vi "Drive Controller.vi"(8 "error in":errorcluster) -> ()   [LabVIEW 2017]
doc: "This VI executes continuously carrying out the current operation and responding to updates or new operation requests. It will often contain the timing or control code that is difficult to place directly in TeleOp. This VI generally opens all sensors and motors and isolates the rest of the robot code from knowing implementation details of how the operations are carried out."
uses:
  <vilib>/Rock Robotics/WPI/SafetyOutput/WPI_SafetyOutputConfigMenu.ctl
  <vilib>/Rock Robotics/WPI/ThirdParty/Sensors/navX/_TypeDefs/FRIC_navX_DeviceNumbersTypeDef.ctl
  <vilib>/addons/control/pid/NI_PID_pid.lvlib
  <vilib>/addons/control/pid/pid.llb/PID (DBL).vi
  <vilib>/Rock Robotics/SystemInterfaces/DIO/FPGA_DIOPWMChannel.ctl
  <vilib>/Rock Robotics/WPI/Counter/WPI_CounterDigitalInputToDigitalSource.vi
  <vilib>/Rock Robotics/SystemInterfaces/DIO/FPGA_DIOChannel.ctl
  Dawgma Programming Library/Controls/PurePursuit/RobotNeededPathData.ctl
  Drive Operations.ctl
  Drive Setpoints.ctl
  Configuration/Constants.vi
  Drive Published Globals.vi
  Framework/Robot Global Data.vi
  <vilib>/Rock Robotics/WPI/DriverStation/WPI_DriverStationRobotMode2.ctl
  <extravilib>/ChannelInstances/Lossy Stream-c(dbl,dbl,dbl,c(dbl,dbl)).lvlib
  <vilib>/Rock Robotics/Network Tables/NT Write Number.vi
  <vilib>/Rock Robotics/SystemInterfaces/i2clib/i2c_bus.ctl
  <vilib>/Rock Robotics/Network Tables/NT Read Number.vi
  <vilib>/Rock Robotics/WPI/RobotDrive/WPI_RobotDriveOpen2MotorWithSPARK.vi
  <vilib>/Rock Robotics/WPI/RobotDrive/WPI_RobotDriveOpen4MotorWithSPARK.vi
  <vilib>/Rock Robotics/WPI/Framework/Completion Status.ctl
panel:
  in  "MaxAccelDistance":dbl=170.0
  in  "MaxVelDistance":dbl=140.0
  in  "MaxAccelAngle":dbl
  in  "MaxVelAngle":dbl
  in  "TurnToAngleGains":T1={"FFV"=0.0032, "FFA"=0.0, "Vel PID"={"P"=0.0, "I"=0.0, "D"=0.0}} {"Vel PID"."D" format="%.3f"; "Vel PID"."I" format="%.3f"; "Vel PID"."P" format="%.3f"}
  in  "PixyCenteringValues":cluster{"X":dbl, "Y":dbl}[](array[cluster])=[{"X"=0.0, "Y"=70.0}, {"X"=70.0, "Y"=100.0}]
  in  "EndCondArea":i32=11000
  in  "MaxY":i32=130
  in  "KpY":dbl=0.0001
  in  "KpX":dbl=0.1
  in  "MaxSpeed":dbl=0.3
  in  "KdX":dbl=0.07
  in  "AreaSetpoint":i32
  in  "CenterSetpoint":i32=80
  out "Numeric":dbl=4.0
  out "Yaw 2":dbl=-45.089999999999996
  in  "Gains":T1={"FFV"=0.0059, "FFA"=0.0019, "Vel PID"={"P"=0.01, "I"=0.0, "D"=0.0}}
  in  "Interactive Values":T2={"Operation"=enum."Turn to Angle", "Left Speed"=-0.27, "Right Speed"=0.27, "Duration"=2.0, "Speed"=0.0, "Start Angle"=0.0, "Target Angle"=180.0, "Distance (inch)"=0.0, "Start Point (inch)"=0.0, "RobotNeededPathData"={"Path"=[], "MaxVel"=0.0, "MaxAccel"=-1.0, "Backwards?"=FALSE, "PointSpacing"=0.0, "LookaheadDist"=0.0, "Speed/Curve"=1.8, "SlowDistanceAtEnd"=12.0, "SlowSpeed"=15.0, "MaxDeAccel"=0.0}, "Start Point 2"=0.0} {"RobotNeededPathData"."SlowSpeed" format="%#_13g"; "RobotNeededPathData"."SlowDistanceAtEnd" format="%#_13g"; "RobotNeededPathData"."Speed/Curve" format="%#_13g"}
  in  "Buttons":cluster{"Execute Cmd":bool, "Abort Cmd":bool}
  out "Command Timing":cluster{"Start Time (ms)":u32, "Iterations":i32}={"Start Time (ms)"=372507, "Iterations"=0}
  out "Status":T5
  out "Setpoints":T6(graph)
  out "Current\nCmd":string="Started at  14:51:47.884\nDefault: Reserve,  L 0.0, R 0.0, D 0.000000"
  # "Tip: The graph shows the motor setpoints. It may also be helpful to observe inputs and sensor values.\nYou may also want to display tuning or debugging controls."
  # ".0088"
  # ".0017"
  # ".02"
  # "Interactive Command: You may fill in the settings for a command\nand schedule it with the Execute button. You can observe and abort\nany command while fine tuning the code for the controller."
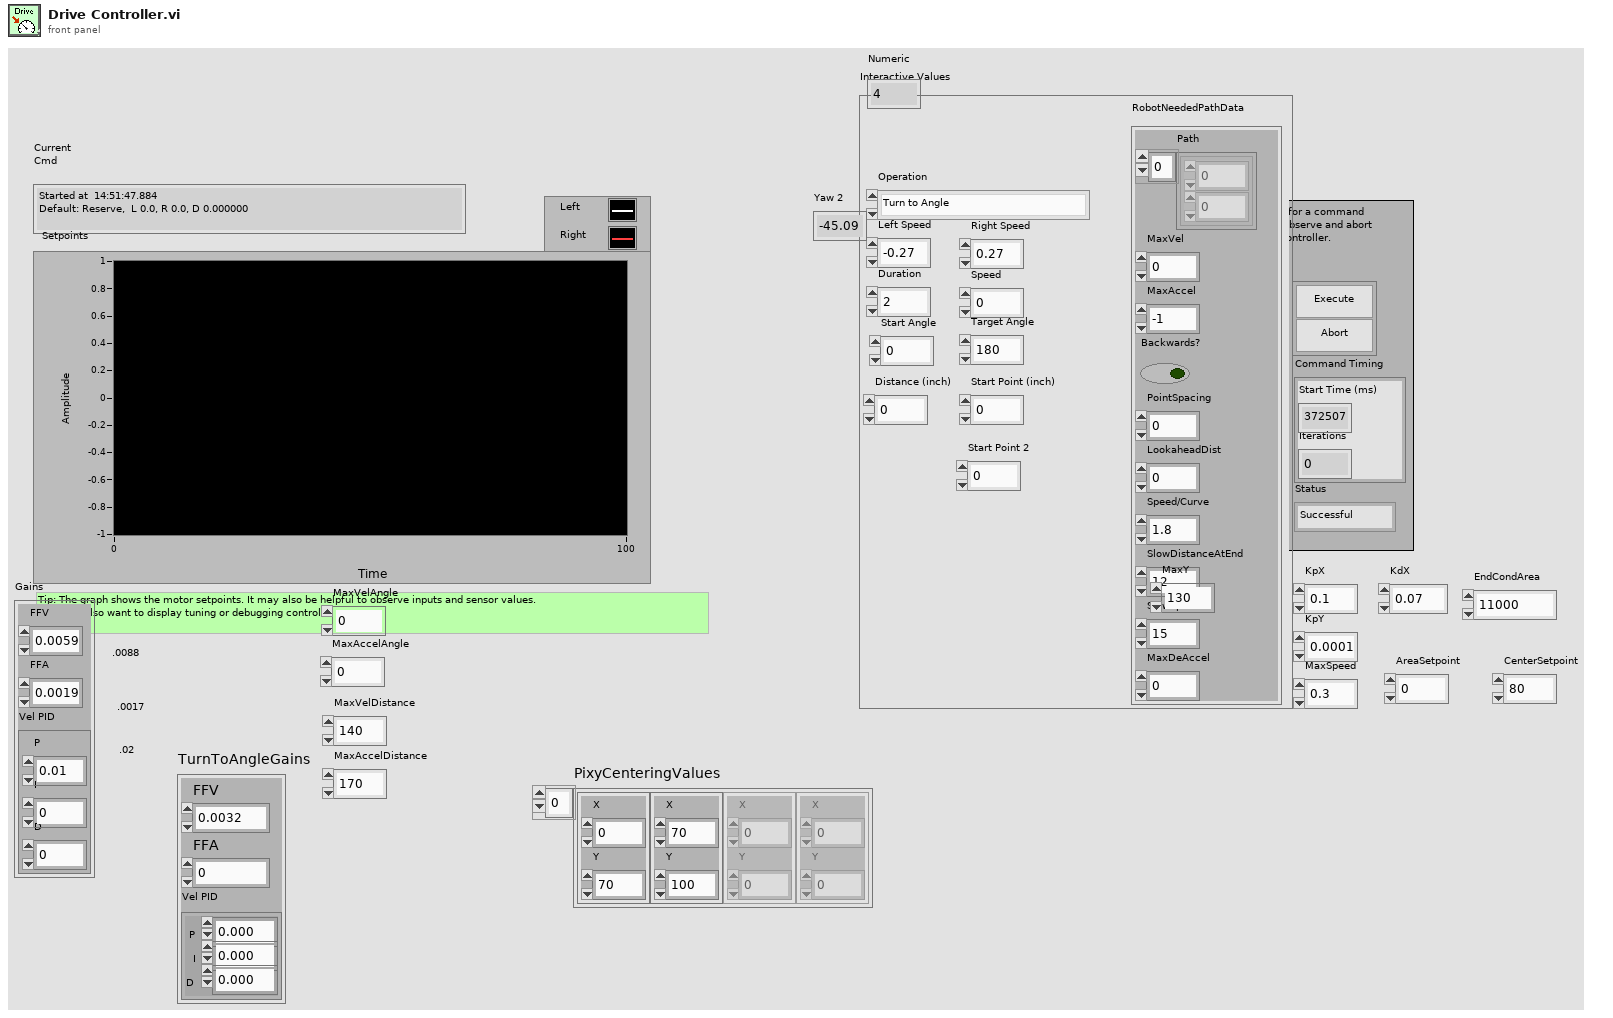
[diagram p1: front panel]
types:
  T1 = cluster{"FFV":dbl, "FFA":dbl, "Vel PID":cluster{"P":dbl, "I":dbl, "D":dbl}}
  T2 = typedef "Drive Setpoints.ctl" = cluster{"Operation":T3, "Left Speed":dbl, "Right Speed":dbl, "Duration":dbl, "Speed":dbl, "Start Angle":dbl, "Target Angle":dbl, "Distance (inch)":dbl, "Start Point (inch)":dbl, "RobotNeededPathData":T4, "Start Point 2":dbl}
  T3 = typedef "Drive Operations.ctl" = enum16{"Reserve", "Read Current", "Immediate", "Drive for Time", "Drive for Distance", "Turn to Angle", "Arc Turn", "Drive Path", "Drive To Cube"}
  T4 = typedef "RobotNeededPathData.ctl" = cluster{"Path":cluster{dbl, dbl}[], "MaxVel":dbl, "MaxAccel":dbl, "Backwards?":bool, "PointSpacing":dbl, "LookaheadDist":dbl, "Speed/Curve":dbl, "SlowDistanceAtEnd":dbl, "SlowSpeed":dbl, "MaxDeAccel":dbl}
  T5 = typedef "Completion Status.ctl" = enum16{"Successful", "Aborted", "Incomplete"}
  T6 = cluster{"Left Setpoint":dbl, "Right Setpoint":dbl}
  T7 = typedef "i2c_bus.ctl" = enum16{"I2C On-Board", "I2C MXP", "Invalid"}
  T8 = typedef "FPGA_DIOChannel.ctl" = enum8{"DIO 0", "DIO 1", "DIO 2", "DIO 3", "DIO 4", "DIO 5", "DIO 6", "DIO 7", "DIO 8", "DIO 9", "DIO MXP 0", "DIO MXP 1", "DIO MXP 2", "DIO MXP 3", "DIO MXP 4", "DIO MXP 5", "DIO MXP 6", "DIO MXP 7", "DIO MXP 8", "DIO MXP 9", "DIO MXP 10", "DIO MXP 11", "DIO MXP 12", "DIO MXP 13", "DIO MXP 14", "DIO MXP 15", "SPI Port CS1", "SPI Port CS2", "SPI Port CS3", "SPI Port MISO", "SPI Port MOSI", "Invalid"}
  T9 = typedef "FPGA_DIOPWMChannel.ctl" = enum8{"PWM 0", "PWM 1", "PWM 2", "PWM 3", "PWM 4", "PWM 5", "PWM 6", "PWM 7", "PWM 8", "PWM 9", "PWM MXP 0", "PWM MXP 1", "PWM MXP 2", "PWM MXP 3", "PWM MXP 4", "PWM MXP 5", "PWM MXP 6", "PWM MXP 7", "PWM MXP 8", "PWM MXP 9", "Invalid"}
  T10 = typedef "WPI_SafetyOutputConfigMenu.ctl" = enum16{"Enable", "Disable"}
  T11 = typedef "WPI_DigitalInputDevRef.ctl" = cluster{"DevStatus":errorcluster, "DIO Channel":T8}
  T12 = typedef "FPGA_CounterEncoderSourceConvertionLVSourceType.ctl" = cluster{"DevStatus":errorcluster, "AnalogTriggerMode?":bool, "DigitalMode":cluster{"DIO Channel":T13}, "AnalogTriggerMode":cluster{"AnalogTriggerIndex":T14, "OutputType":T15}}
  T13 = typedef "FPGA_DIODigitalSourceChannel.ctl" = enum8{"DIO 0", "DIO 1", "DIO 2", "DIO 3", "DIO 4", "DIO 5", "DIO 6", "DIO 7", "DIO 8", "DIO 9", "DIO MXP 0", "DIO MXP 1", "DIO MXP 2", "DIO MXP 3", "DIO MXP 4", "DIO MXP 5", "DIO MXP 6", "DIO MXP 7", "DIO MXP 8", "DIO MXP 9", "DIO MXP 10", "DIO MXP 11", "DIO MXP 12", "DIO MXP 13", "DIO MXP 14", "DIO MXP 15", "Disabled"}
  T14 = typedef "FPGA_AnalogTriggerIndex.ctl" = enum8{"Trig 0", "Trig 1", "Trig 2", "Trig 3", "Trig 4", "Trig 5", "Trig 6", "Trig 7", "Invalid"}
  T15 = typedef "FPGA_AnalogTriggerOutType.ctl" = enum16{"InWindow", "TriggerState", "Rising", "Falling"}
  T16 = typedef "WPI_EncoderDevRef.ctl" = cluster{"DevStatus":errorcluster, "EncoderIndex":T17, "CounterIndex":T18, "DistancePerCount":dbl, "Decoding Type":T19}
  T17 = typedef "FPGA_EncoderIdx.ctl" = enum8{"Enc 0", "Enc 1", "Enc 2", "Enc 3", "Enc 4", "Enc 5", "Enc 6", "Enc 7", "Invalid"}
  T18 = typedef "FPGA_CounterCtrSystemIndex.ctl" = enum8{"Ctr 0", "Ctr 1", "Ctr 2", "Ctr 3", "Ctr 4", "Ctr 5", "Ctr 6", "Ctr 7", "Invalid"}
  T19 = typedef "WPI_EncoderType.ctl" = enum16{"1x", "2x", "4x"}
  T20 = typedef "WPI_RobotDriveDevRef.ctl" = cluster{"DevStatus":errorcluster, "Motors[]":T21[], "Square Inputs":bool, "Max Output":dbl}
  T21 = typedef "WPI_MotorControlDeviceRef.ctl" = cluster{"DeviceStatus":errorcluster, "Type":T22, "PWM":cluster{"PWM Channel":T9, "DeadBand":T23}, "CAN":cluster{"Device Number":u8, "SetOutput VI Ref":variant, "GetOutput VI Ref":variant, "Enable VI Ref":variant, "Disable VI Ref":variant, "Data":variant}, "Invert":bool, "DIO PWM":cluster{"PWM \"Enable\" Channel":T9, "DIOChannel":T8, "PWM Rate":dbl}}
  T22 = typedef "WPI_MotorControlType.ctl" = enum16{"PWM", "CAN", "DIO PWM"}
  T23 = typedef "WPI_PWMDeadband.ctl" = cluster{"Name":string, "maxPositivePwm":i32, "minPositivePwm":i32, "centerPwm":i32, "maxNegativePwm":i32, "minNegativePwm":i32, "angularRange":u16}
  T24 = typedef "WPI_I2CDevRef.ctl" = cluster{"DevStatus":errorcluster, "Device Address":u8, "Handle":i32, "I2C Bus":T7}
  T25 = typedef "Command Status Info.ctl" = cluster{"Name":string, "Status":T5, "notifier out":T26}
  T26 = typedef "Completion Notifier.ctl" = refnum<notifier>
  T27 = cluster{"SubSystem Data":T2, cluster{"Start Time (ms)":u32, "Iterations":i32}, cluster{"Command Info":T25, "Description":string, "Default Command":T2, "queue out":refnum<queue>, "Subsystem Name":string}}
  T28 = cluster{"X":i32, "Y":i32, "Width":i32, "Height":i32, "ValidData":bool, "Timestamp":u32}
  T29 = typedef "WPI_DriverStationRobotMode2.ctl" = enum16{"Autonomous Disabled", "Autonomous Enabled", "Teleop Disabled", "Teleop Enabled", "Disconnected", "Finish", "Test Disabled", "Test Enabled", "Emergency Stopped"}
  T30 = cluster{"Yaw":dbl, "Roll":dbl, "Pitch":dbl, "Heading":dbl, "Fused Heading":dbl}
  T31 = cluster{"dx/dt":dbl, "dx/dt":dbl, dbl, cluster{dbl, dbl}}
  T32 = typedef "Lossy Stream-c(dbl,dbl,dbl,c(dbl,dbl)).lvlib/)Channel.ctl" = refnum<queue>
  T33 = cluster{"LeftDistance":dbl, "RightDistance":dbl, "LeftVelocity":dbl, "RightVelocity":dbl, "Angle":dbl, "Location":cluster{dbl, dbl}}
  T34 = typedef "FRIC_navX_DeviceNumbersTypeDef.ctl" = enum16{"Dev0", "Dev1", "Dev2", "Dev3"}
  T35 = cluster{"proportional gain (Kc)":dbl, "integral time (Ti, min)":dbl, "derivative time (Td, min)":dbl}
  T36 = cluster{"dx/dt":dbl, "dx/dt":dbl, "Yaw":dbl, cluster{dbl, dbl}}
  T37 = cluster{"SubSystem Data":T2, cluster{"Start Time (ms)":u32, "Iterations":i32}, "Default Command Arguments":cluster{"Command Info":T25, "Description":string, "Default Command":T2, "queue out":refnum<queue>, "Subsystem Name":string}}
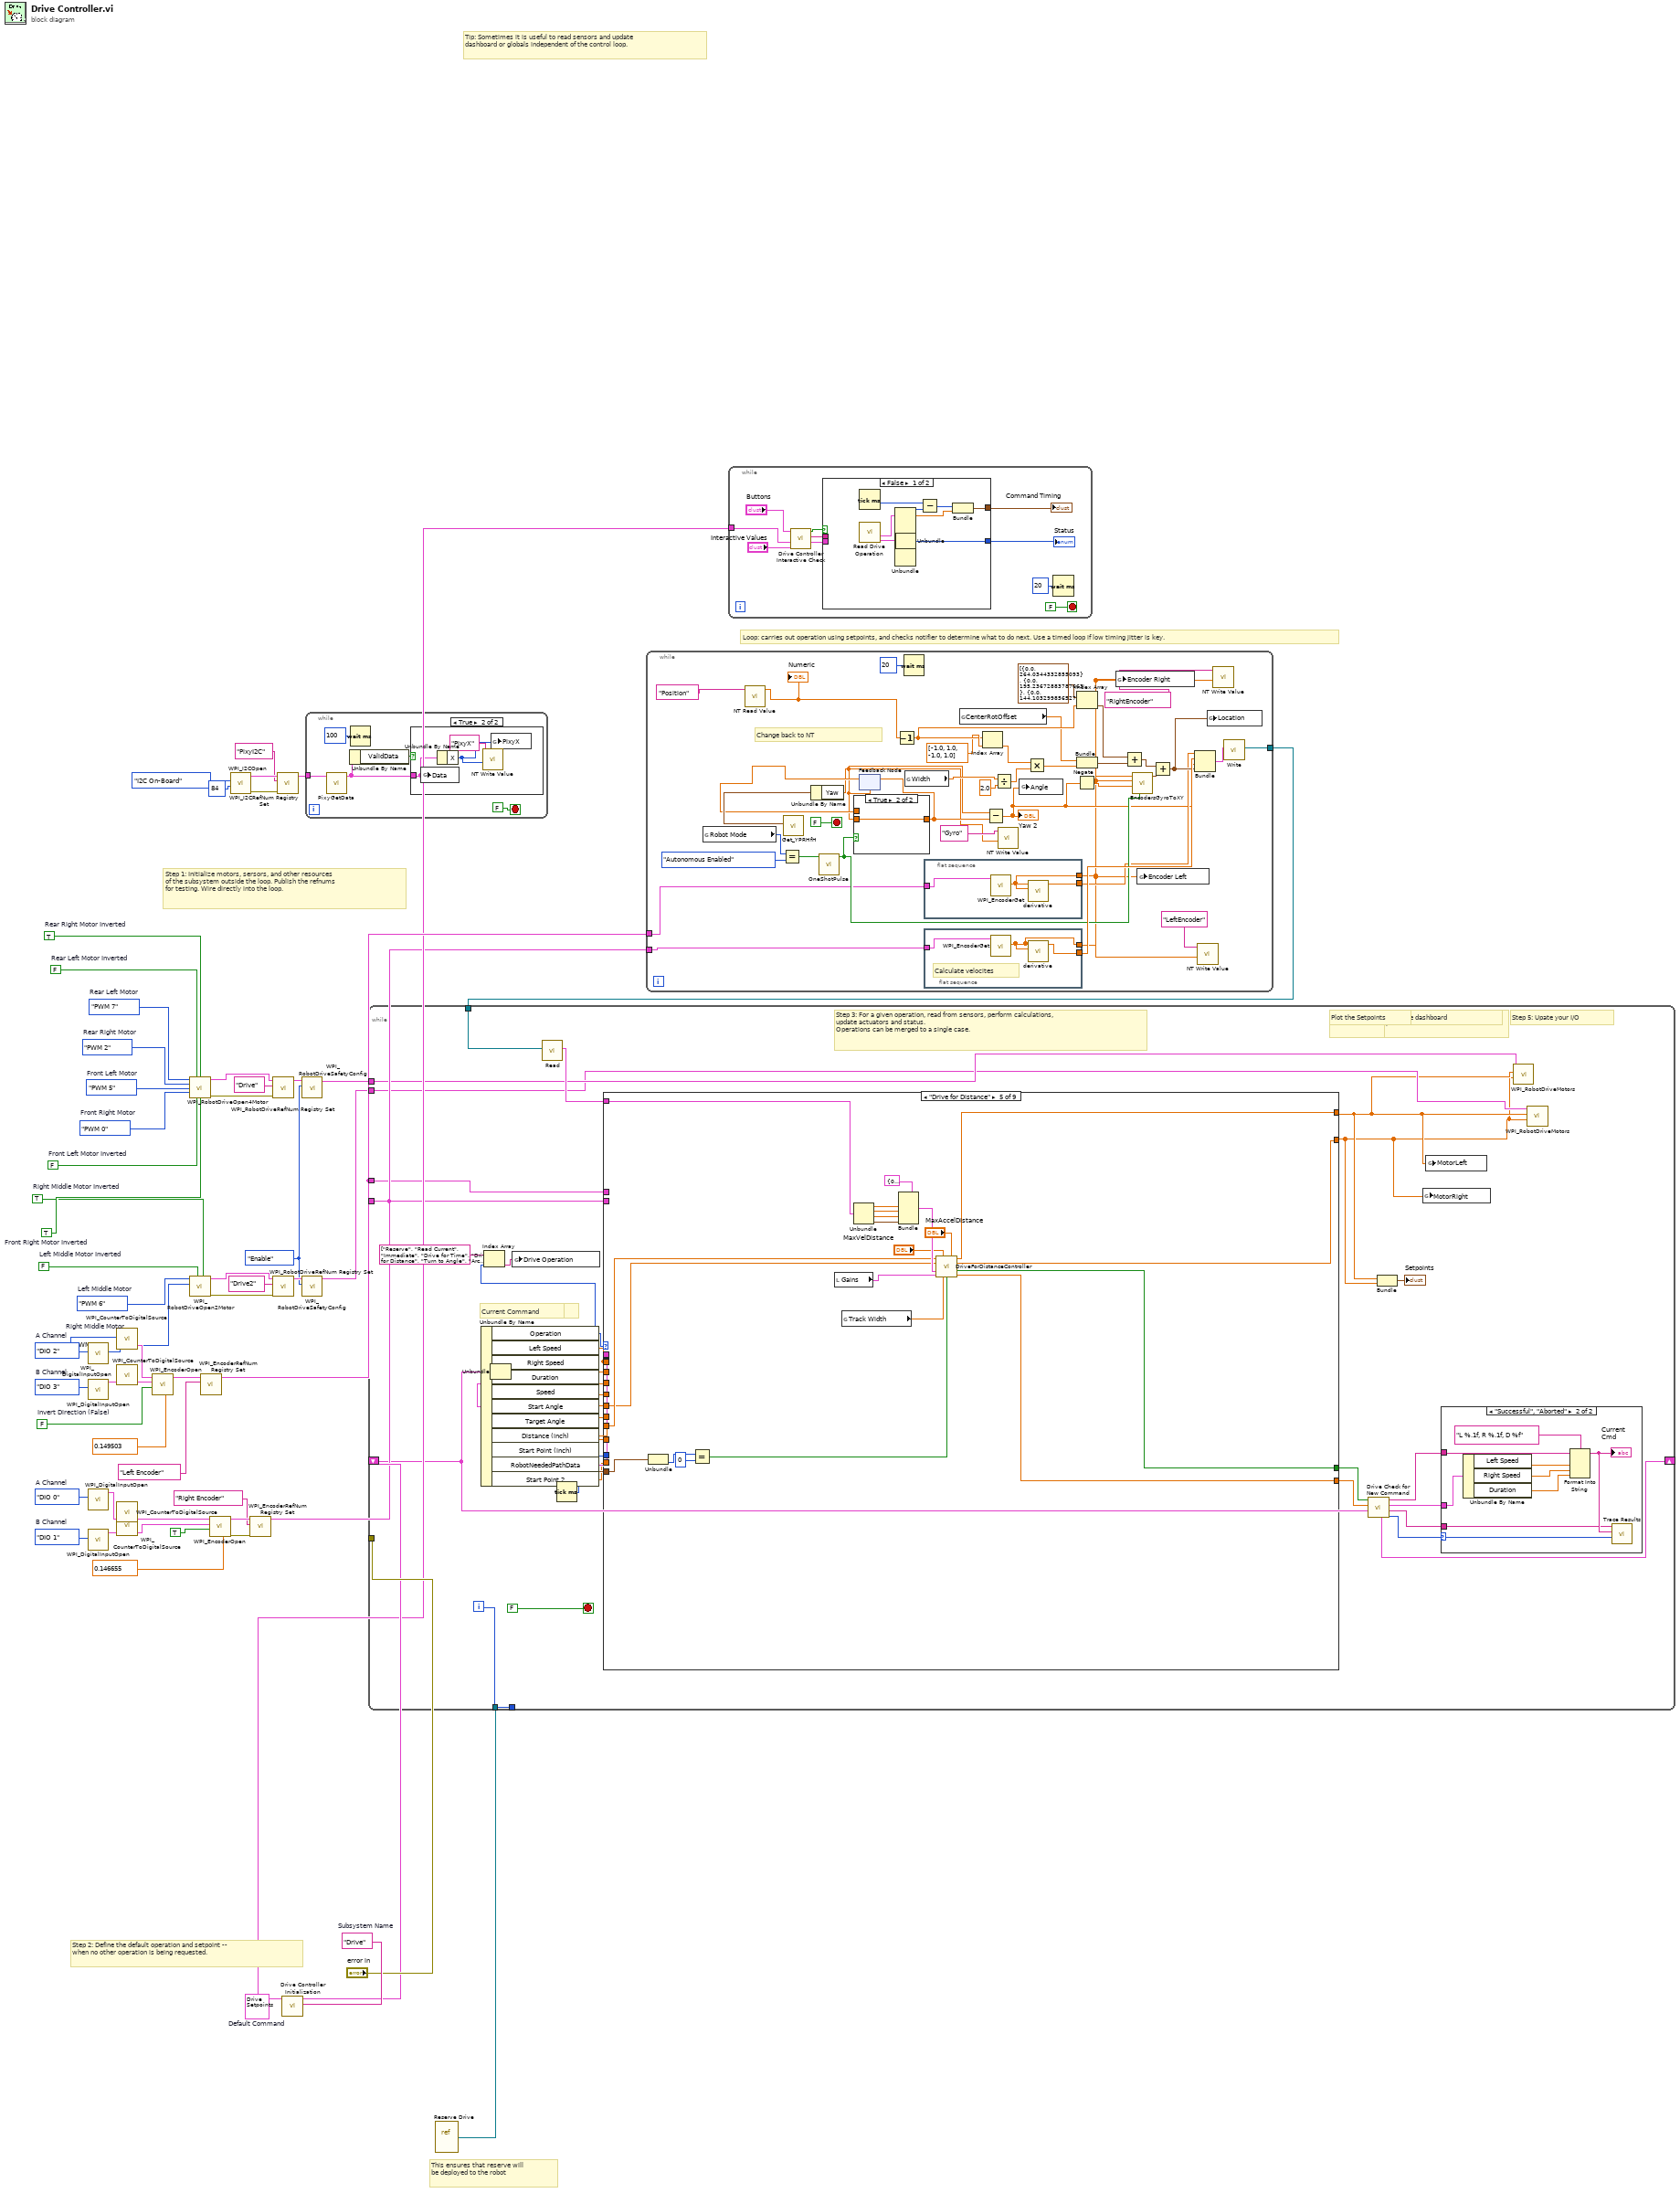
[diagram p0: block diagram]
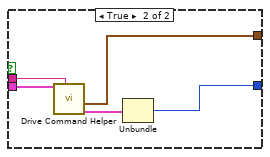
[diagram p4: hidden frame]
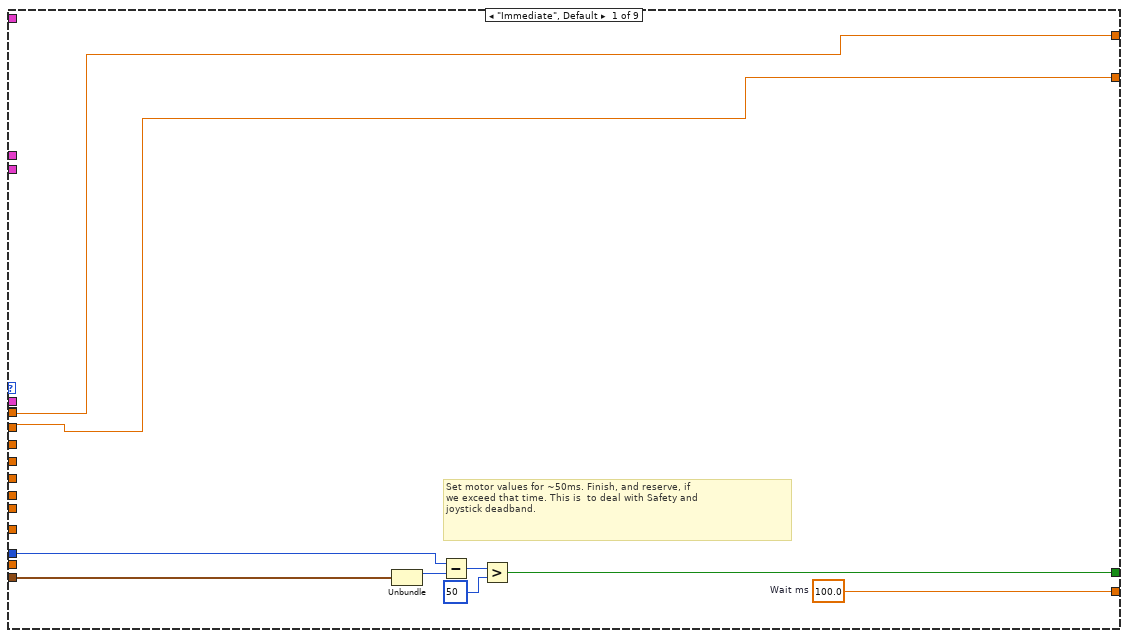
[diagram p5: hidden frame]
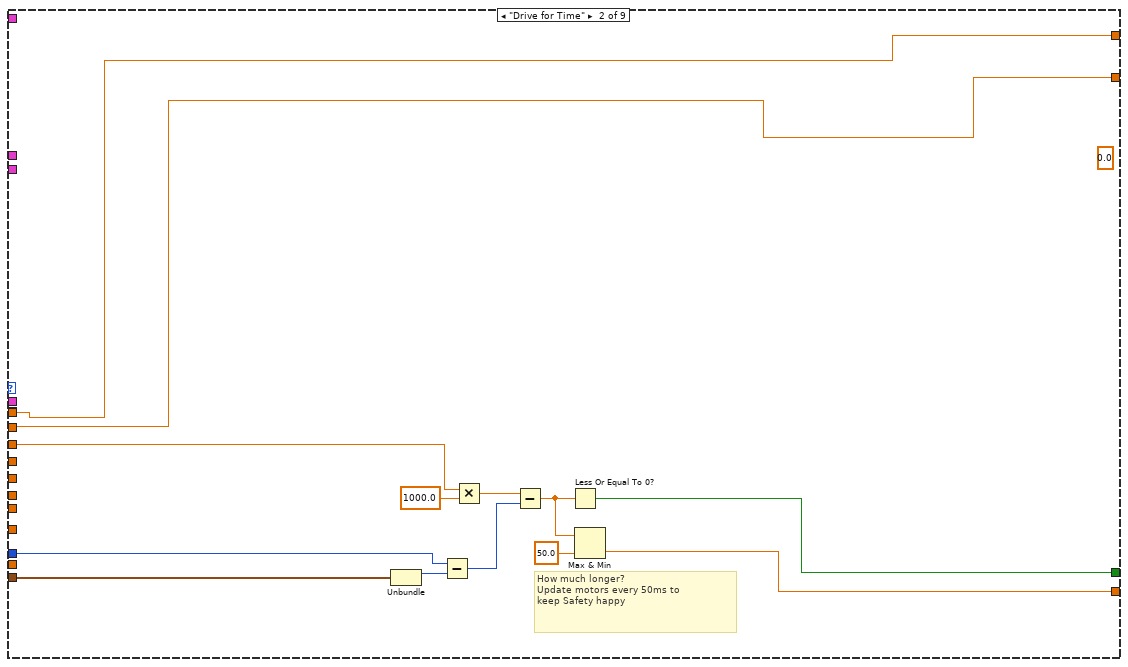
[diagram p6: hidden frame]
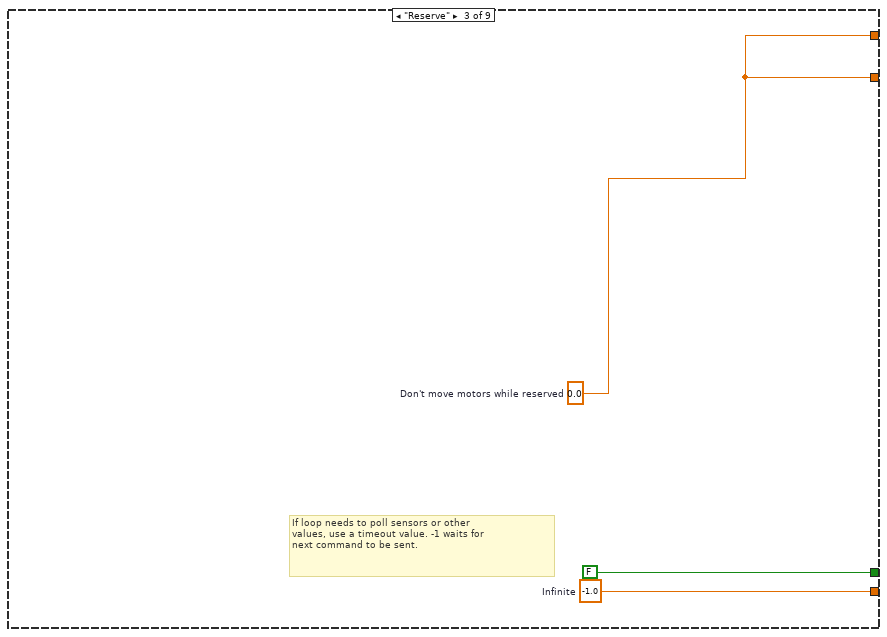
[diagram p7: hidden frame]
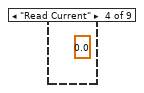
[diagram p8: hidden frame]
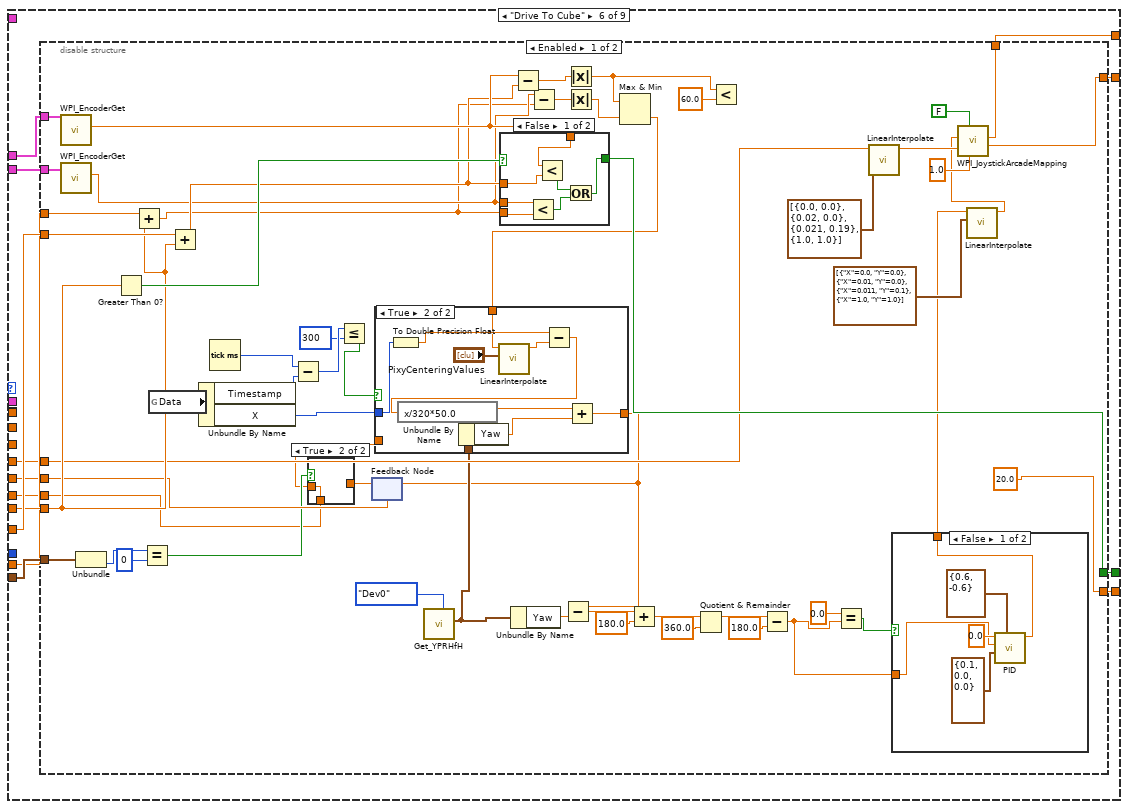
[diagram p9: hidden frame]
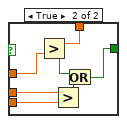
[diagram p12: hidden frame]
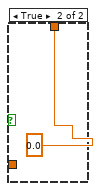
[diagram p13: hidden frame]
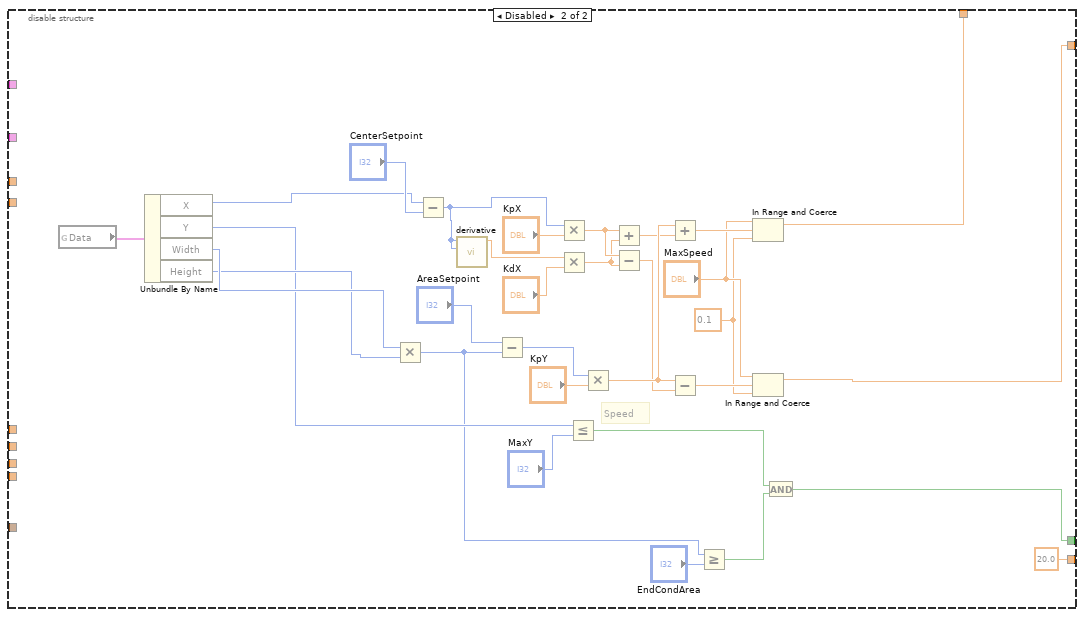
[diagram p14: hidden frame]
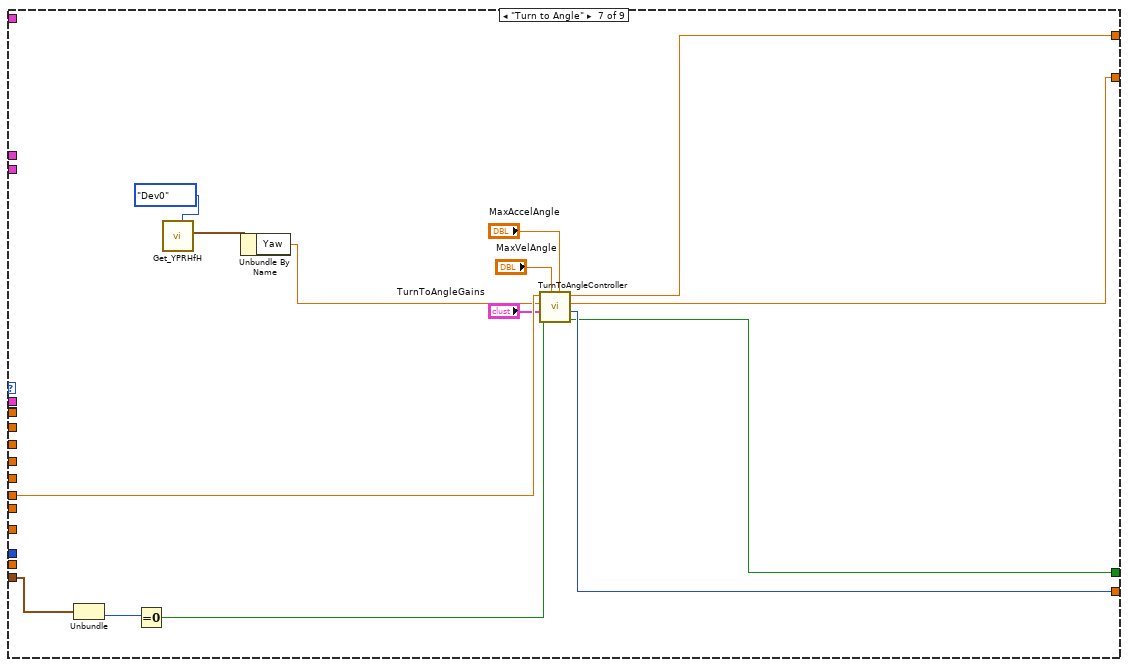
[diagram p15: hidden frame]
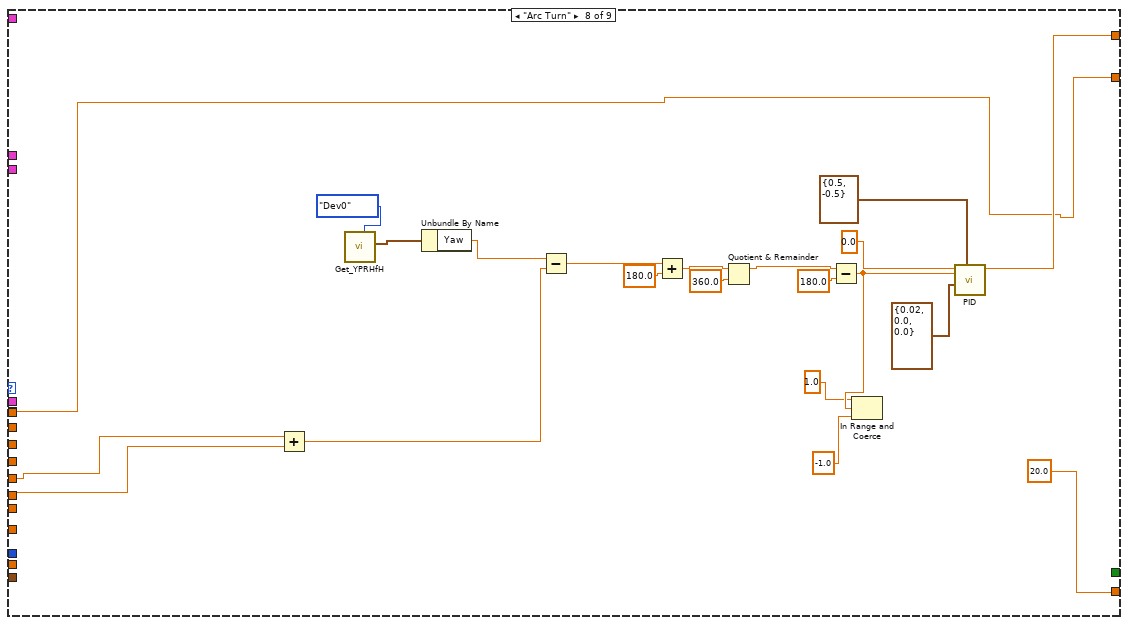
[diagram p16: hidden frame]
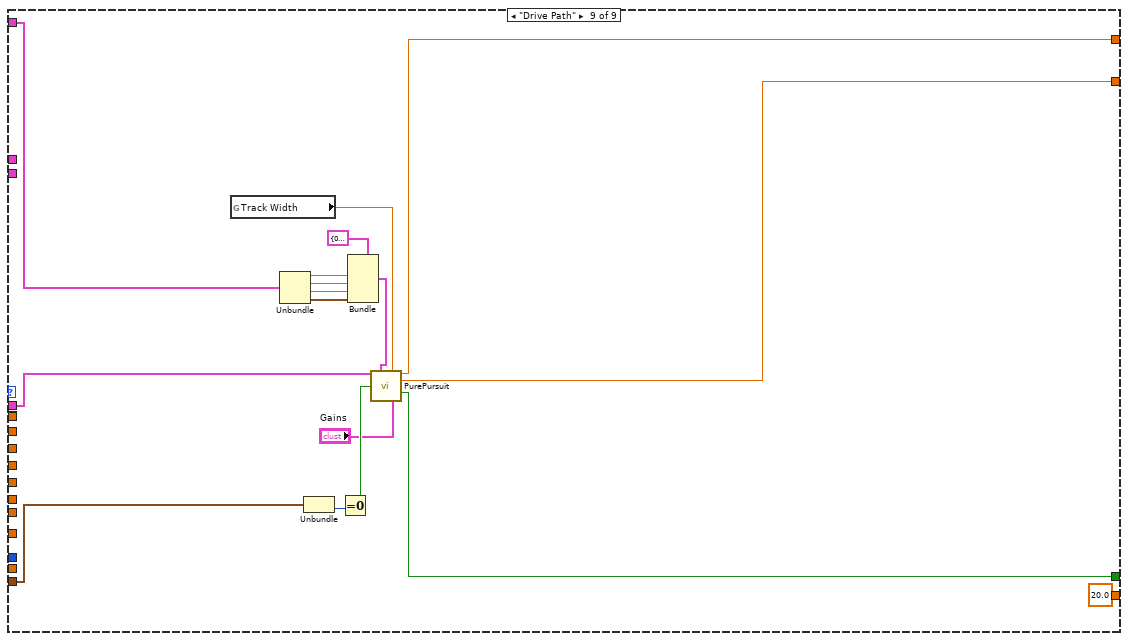
[diagram p17: hidden frame]
diagram:
  w10 = FPGA_DIOChannel."DIO 1"  # B Channel
  w13 = FPGA_DIOChannel."DIO 0"  # A Channel
  w20 = T2 {"Operation"=enum."Reserve", "Left Speed"=0.0, "Right Speed"=0.0, "Duration"=0.0, "Speed"=0.0, "Start Angle"=0.0, "Target Angle"=0.0, "Distance (inch)"=0.0, "Start Point (inch)"=0.0, "RobotNeededPathData"={"Path"=[], "MaxVel"=0.0, "MaxAccel"=0.0, "Backwards?"=FALSE, "PointSpacing"=0.0, "LookaheadDist"=0.0, "Speed/Curve"=1.8, "SlowDistanceAtEnd"=12.0, "SlowSpeed"=15.0, "MaxDeAccel"=0.0}, "Start Point 2"=0.0}  # Default Command
  w27 = TRUE  # Right Middle Motor Inverted
  w28 = FALSE  # Left Middle Motor Inverted
  w31 = FPGA_DIOPWMChannel."PWM 1"  # Right Middle Motor
  w32 = FPGA_DIOPWMChannel."PWM 6"  # Left Middle Motor
  w41 = FALSE  # Invert Direction (False)
  w34 = FPGA_DIOChannel."DIO 3"  # B Channel
  w35 = FPGA_DIOChannel."DIO 2"  # A Channel
  w43 = TRUE  # Front Right Motor Inverted
  w44 = FALSE  # Front Left Motor Inverted
  w45 = TRUE  # Rear Right Motor Inverted
  w46 = FALSE  # Rear Left Motor Inverted
  w47 = FPGA_DIOPWMChannel."PWM 0"  # Front Right Motor
  w48 = FPGA_DIOPWMChannel."PWM 5"  # Front Left Motor
  w49 = FPGA_DIOPWMChannel."PWM 2"  # Rear Right Motor
  w50 = FPGA_DIOPWMChannel."PWM 7"  # Rear Left Motor
  w22 = WPI_SafetyOutputConfigMenu."Enable" ("mode")
  w58 = "Drive"  # Subsystem Name
  # "Step 1: Initialize motors, sersors, and other resources\nof the subsystem outside the loop. Publish the refnums\nfor testing. Wire directly into the loop."
  # "Step 2: Define the default operation and setpoint --\nwhen no other operation is being requested."
  # "This ensures that reserve will\nbe deployed to the robot"
  # "Tip: Sometimes it is useful to read sensors and update\ndashboard or globals independent of the control loop."
  # "Loop: carries out operation using setpoints, and checks notifier to determine what to do next. Use a timed loop if low timing jitter is key."
  n1 = call <vilib>:"WPI_DigitalInputOpen.vi"("DIO Channel"=w35) -> ("DigitalInputDevRef"=w38:T11)  [unwired: 1 in, 9 out]
  n2 = call <vilib>:"WPI_DigitalInputOpen.vi"("DIO Channel"=w34) -> ("DigitalInputDevRef"=w37:T11)  [unwired: 1 in, 9 out]
  n3 = call <vilib>:"WPI_DigitalInputOpen.vi"("DIO Channel"=w13) -> ("DigitalInputDevRef"=w14:T11)  [unwired: 1 in, 9 out]
  n4 = call <vilib>:"WPI_DigitalInputOpen.vi"("DIO Channel"=w10) -> ("DigitalInputDevRef"=w11:T11)  [unwired: 1 in, 9 out]
  n5 = call-poly <vilib>:"WPI_CounterToDigitalSource.vi"("DigitalInputDevRef"=w38) -> ("Digital Source"=w39:T12)  [unwired: 6 out]
  n6 = call-poly <vilib>:"WPI_CounterToDigitalSource.vi"("DigitalInputDevRef"=w37) -> ("Digital Source"=w36:T12)  [unwired: 6 out]
  n7 = call-poly <vilib>:"WPI_CounterToDigitalSource.vi"("DigitalInputDevRef"=w14) -> ("Digital Source"=w15:T12)  [unwired: 6 out]
  n8 = call-poly <vilib>:"WPI_CounterToDigitalSource.vi"("DigitalInputDevRef"=w11) -> ("Digital Source"=w12:T12)  [unwired: 6 out]
  n9 = call <vilib>:"WPI_EncoderOpen.vi"("DistancePerCount"=0.149503, "Invert Direction (False)"=w41, "BSource"=w36, "ASource"=w39) -> ("EncoderDevRef"=w40:T16)  [unwired: 4 in, 3 out]
  n10 = call-poly <vilib>:"WPI_RobotDriveOpen4Motor.vi"("Rear Left Motor"=w50, "Rear Left Motor Inverted"=w46, "Rear Right Motor Inverted"=w45, "Rear Right Motor"=w49, "Front Left Motor"=w48, "Front Right Motor"=w47, "Front Left Motor Inverted"=w44, "Front Right Motor Inverted"=w43) -> ("RobotDriveDevRef"=w57:T20, "error out"=w55:errorcluster)  [unwired: 6 in]
  n11 = call-poly <vilib>:"WPI_RobotDriveOpen2Motor.vi"("Right Motor Inverted"=w27, "Left Motor Inverted"=w28, "Right Motor"=w31, "Left Motor"=w32) -> ("error out"=w26:errorcluster, "RobotDriveDevRef"=w30:T20)  [unwired: 6 in]
  n12 = call <vilib>:"WPI_EncoderRefNum Registry Set.vi"("refnum name"="Left Encoder", "EncoderDevRef"=w40) -> ("EncoderDevRef"=w33:T16)  [unwired: 8 in, 1 out]
  n13 = call <vilib>:"WPI_EncoderOpen.vi"("DistancePerCount"=0.146655, "Invert Direction (False)"=TRUE, "BSource"=w12, "ASource"=w15) -> ("error out"=w17:errorcluster, "EncoderDevRef"=w16:T16)  [unwired: 4 in, 2 out]
  n14 = call <vilib>:"WPI_I2COpen.vi"("Device Address"=u8 84, "I2C Bus"=i2c_bus."I2C On-Board") -> ("error out"=w3:errorcluster, "I2CDevRef"=w4:T24)  [unwired: 8 in]
  n15 = call <vilib>:"WPI_EncoderRefNum Registry Set.vi"("error in (no error)"=w17, "refnum name"="Right Encoder", "EncoderDevRef"=w16) -> ("EncoderDevRef"=w18:T16)  [unwired: 7 in, 1 out]
  n16 = call <vilib>:"WPI_RobotDriveRefNum Registry Set.vi"("error in (no error)"=w55, "refnum name"="Drive", "RobotDriveDevRef"=w57) -> ("RobotDriveDevRef"=w25:T20)  [unwired: 1 in, 7 out]
  n17 = call <vilib>:"WPI_RobotDriveRefNum Registry Set.vi"("error in (no error)"=w26, "refnum name"="Drive2", "RobotDriveDevRef"=w30) -> ("RobotDriveDevRef"=w24:T20)  [unwired: 7 in, 1 out]
  n18 = call <vilib>:"WPI_I2CRefNum Registry Set.vi"("error in (no error)"=w3, "refnum name"="PixyI2C", "I2CDevRef"=w4) -> ("I2CDevRef"=w1:T24)  [unwired: 7 in, 1 out]
  n19 = call "Drive Controller Initialization.vi"("Subsystem Name"=w58, "Default Command"=w20) -> ("Current Command"=w52:T27)  [unwired: 9 in]
  n20 = call <vilib>:"WPI_RobotDriveSafetyConfig.vi"("mode"=w22, "RobotDriveDevRef"=w25) -> ("RobotDriveDevRef"=w54:T20)  [unwired: 8 in, 1 out]
  n21 = call <vilib>:"WPI_RobotDriveSafetyConfig.vi"("mode"=w22, "RobotDriveDevRef"=w24) -> ("RobotDriveDevRef"=w23:T20)  [unwired: 8 in, 1 out]
  n22 = while {
    tunnel: w1 -> [w62]
    stop <- FALSE stop-if-true
    n23 = call "PixyGetData.vi"("I2CDevRef"=w62) -> ("Data"=w61:T28)  [unwired: 10 in]
    n24 = Unbundle By Name(w61) -> ("ValidData"=w60:bool)
    n25 = Wait (ms)(milliseconds to wait=u32 100) -> ()  [unwired: 1 out]
    n26 = case shown="True" w60 {
      tunnel: w61 -> [_ w66]
      frame False {
      }
      frame True {
        n27 = global write "Drive Published Globals.vi" "Data"(w66) -> ()
        n28 = Unbundle By Name(w66) -> ("X"=w64:i32)
        n29 = call-poly <vilib>:"NT Write Value.vi"("Numeric"=w64, "Name"="PixyX") -> ()  [unwired: 9 in, 1 out]
        n30 = global write "Drive Published Globals.vi" "PixyX"(w64) -> ()
      }
    }
  }
  n31 = vi-ref "Reserve Drive.vi"() -> (w51:refnum<vi>)
  n32 = while {
    tunnel: [w78] -> w19
    tunnel: w18 -> [w77]
    tunnel: w33 -> [w76]
    stop <- FALSE stop-if-true
    # "Change back to NT"
    n33 = global read "Robot Global Data.vi" "Robot Mode"() -> (w93:T29)
    n34 = call-poly <vilib>:"NT Read Value.vi"("Name"="Position") -> ("Numeric"=w74:dbl)  [unwired: 9 in, 1 out]
    "Numeric" <- w74
    n35 = Equal?(x=w93, y=WPI_DriverStationRobotMode2."Autonomous Enabled") -> (x = y?=w94:bool)
    n36 = call <vilib>:"Get_YPRHfH.vi"() -> ("YRPHfH"=w105:T30)  [unwired: 11 in]
    n37 = Unbundle By Name(w105) -> ("Yaw"=w67:dbl)
    n38 = call "OneShotPulse.vi"("Input"=w94) -> ("Output"=w95:bool)  [unwired: 10 in]
    n39 = feedback #1(w67) -> (w96:dbl)
    n40 = case shown="True" w95 {
      tunnel: w67 -> [_ w110]
      tunnel: [w109 w110] -> w97
      tunnel: w96 -> [w109 _]
      frame False {
      }
      frame True {
      }
    }
    n41 = feedback-in #1(w97) -> ()
    n42 = Decrement(x=w74) -> (x-1=w87:dbl)
    n43 = Wait (ms)(milliseconds to wait=u32 20) -> ()  [unwired: 1 out]
    n44 = global read "Constants.vi" "Width"() -> (w82:dbl)
    n45 = flat-sequence {
      tunnel: [w108] -> w79
      tunnel: [w107] -> w70
      tunnel: w76 -> [w106]
      frame #0 {
        n46 = call <vilib>:"WPI_EncoderGet.vi"("EncoderDevRef"=w106) -> ("Distance"=w107:dbl)  [unwired: 5 in, 5 out]
        n47 = call "derivative.vi"("Starting value"=w107, "x"=w107) -> ("dx/dt"=w108:dbl)  [unwired: 9 in]
      }
    }
    n48 = flat-sequence {
      tunnel: [w112] -> w102
      tunnel: [w111] -> w68
      tunnel: w77 -> [w113]
      frame #0 {
        # "Calculate velocites"
        n49 = call <vilib>:"WPI_EncoderGet.vi"("EncoderDevRef"=w113) -> ("Distance"=w111:dbl)  [unwired: 5 in, 5 out]
        n50 = call "derivative.vi"("Starting value"=w111, "x"=w111) -> ("dx/dt"=w112:dbl)  [unwired: 9 in]
      }
    }
    n51 = global read "Constants.vi" "CenterRotOffset"() -> (w80:dbl)
    n52 = Index Array(array=dbl[] [-1.0, 1.0, -1.0, 1.0], index=w87) -> (element=w88:dbl)
    n53 = Subtract(x=w67, y=w97) -> (x-y=w72:dbl)
    "Yaw 2" <- w72
    n54 = Divide(x=w82, y=2.0) -> (x/y=w83:dbl)
    n55 = call-poly <vilib>:"NT Write Value.vi"("Numeric"=w67, "Name"="Gyro") -> ()  [unwired: 9 in, 1 out]
    n56 = global write "Drive Published Globals.vi" "Angle"(w72) -> ()
    n57 = Multiply(x=w88, y=w83) -> (x*y=w89:dbl)
    n58 = Negate(x=w72) -> (-x=w98:dbl)
    n59 = Index Array(array=cluster{dbl, dbl}[] [{0.0, 264.0344332855093}, {0.0, 195.23672883787663}, {0.0, 144.10329985652797}, {0.0, -0.0}] ("x*y"), index=w87) -> (element=w86:cluster{dbl, dbl})
    n60 = Bundle("CenterRotOffset"=w80, w89) -> (w90:cluster{"CenterRotOffset":dbl, dbl})  [unwired: 1 in]
    n61 = global write "Drive Published Globals.vi" "Encoder Right"(w68) -> ()
    n62 = Add(x=w86, y=w90) -> (x+y=w91:cluster{dbl, dbl})
    n63 = call "EncodersGyroToXY.vi"("Reset"=w95, "Angle (degrees)"=w98, "Right Distance"=w68, "Left Distance"=w70) -> ("Location"=w99:cluster{dbl, dbl})  [unwired: 7 in]
    n64 = global write "Drive Published Globals.vi" "Encoder Left"(w70) -> ()
    n65 = Add(x=w91, y=w99) -> (x+y=w100:cluster{dbl, dbl})
    n66 = Bundle("dx/dt"=w79, "dx/dt"=w102, w72, w100) -> (w101:T31)  [unwired: 1 in]
    n67 = call-poly <vilib>:"NT Write Value.vi"("Numeric"=w70, "Name"="LeftEncoder") -> ()  [unwired: 9 in, 1 out]
    n68 = global write "Drive Published Globals.vi" "Location"(w100) -> ()
    n69 = call-poly <vilib>:"NT Write Value.vi"("Numeric"=w68, "Name"="RightEncoder") -> ()  [unwired: 9 in, 1 out]
    n70 = call <extravilib>:"Write.vi"("element"=w101) -> ("channel"=w78:T32)  [unwired: 8 in, 2 out]
  }
  n71 = while {
    shift-right: [w144] -> _
    shift-left: w52 -> [w137]
    tunnel: [w147] -> _
    tunnel: w54 -> [w123]
    tunnel: "error in" -> [_]
    tunnel: w51 -> [_]
    tunnel: w33 -> [w121]
    tunnel: w23 -> [w122]
    tunnel: w19 -> [w125]
    tunnel: w18 -> [w120]
    i -> [w147]
    stop <- FALSE stop-if-true
    # "Plot the Setpoints"
    # "Step 5: Upate your I/O"
    # "Step 4: Format a string to describe this\ncmd and how the previous cmd finished"
    # "Current Command"
    # "Update motors and update dashboard"
    # "Access Cmd setpoints"
    # "Finished? &\nWait Time"
    # "Step 3: For a given operation, read from sensors, perform calculations,\nupdate actuators and status.\nOperations can be merged to a single case."
    n72 = Unbundle(w137) -> ("SubSystem Data"=w126:T2, w138:cluster{"Start Time (ms)":u32, "Iterations":i32})  [unwired: 1 out]
    n73 = Unbundle By Name(w126) -> ("Operation"=w116:T3, "Left Speed"=w135:dbl, "Right Speed"=w134:dbl, "Duration"=w133:dbl, "Speed"=w132:dbl, "Start Angle"=w131:dbl, "Target Angle"=w130:dbl, "Distance (inch)"=w129:dbl, "Start Point (inch)"=w128:dbl, "RobotNeededPathData"=w127:T4, "Start Point 2"=w119:dbl)
    n74 = Index Array(array=string[] ["Reserve", "Read Current", "Immediate", "Drive for Time", "Drive for Distance", "Turn to Angle", "Arc Turn", "Drive Path", "Drive To Cube"] ("Strings []"), index=w116) -> (element=w114:string)
    n75 = global write "Robot Global Data.vi" "Drive Operation"(w114) -> ()
    n76 = call <extravilib>:"Read.vi"("channel"=w125) -> ("element"=w124:T36)  [unwired: 5 in, 5 out]
    n77 = Tick Count (ms)() -> (millisecond timer value=w146:u32)
    n78 = case shown="\"Drive for Distance\"" w116 {
      tunnel: [w157 w161 w173 _ w188 w206 w329 20.0 ("Infinite") 20.0 ("Infinite")] -> w143
      tunnel: [w152 w165 FALSE ("ignore previous (F)") _ w189 w207 w328 _ w376] -> w142
      tunnel: w138 -> [w151 w167 _ _ w194 w203 w340 _ w366]
      tunnel: w146 -> [w153 w164 _ _ _ _ _ _ _]
      tunnel: [w150 w159 w171 _ w191 w198 w331 w343 w378] -> w118
      tunnel: [w149 w158 w171 _ w190 w197 w330 w342 w377] -> w117
      tunnel: w132 -> [_ _ _ _ _ w199 _ _ _]
      tunnel: w129 -> [_ _ _ _ w177 w201 _ _ _]
      tunnel: w133 -> [_ w160 _ _ _ _ _ _ _]
      tunnel: w135 -> [w150 _ _ _ _ _ _ w342 _]
      tunnel: w134 -> [w149 w158 _ _ _ _ _ _ _]
      tunnel: w121 -> [_ _ _ _ _ w205 _ _ _]
      tunnel: w131 -> [_ _ _ _ w176 w196 _ w346 _]
      tunnel: w130 -> [_ _ _ _ _ w195 w338 w345 _]
      tunnel: w128 -> [_ _ _ _ _ w204 _ _ _]
      tunnel: w135 -> [_ w159 _ _ _ _ _ _ _]
      tunnel: w127 -> [_ _ _ _ _ _ _ _ w379]
      tunnel: w124 -> [_ _ _ _ w181 _ _ _ w370]
      tunnel: w120 -> [_ _ _ _ _ w202 _ _ _]
      tunnel: w119 -> [_ _ _ _ _ w200 _ _ _]
      frame "Immediate", Default {
        w157 = 100.0  # Wait ms
        # "Set motor values for ~50ms. Finish, and reserve, if\nwe exceed that time. This is  to deal with Safety and\njoystick deadband."
        n79 = Unbundle(w151) -> ("Start Time (ms)"=w154:u32)  [unwired: 1 out]
        n80 = Subtract(x=w153, y=w154) -> (x-y=w155:u32)
        n81 = Greater?(x=w155, y=u8 50 ("Left Motor")) -> (0:w152:bool)
      }
      frame "Drive for Time" {
        (unwired) 0.0 ("output")
        # "How much longer?\nUpdate motors every 50ms to\nkeep Safety happy"
        n82 = Unbundle(w167) -> ("Start Time (ms)"=w166:u32)  [unwired: 1 out]
        n83 = Subtract(x=w164, y=w166) -> (x-y=w170:u32)
        n84 = Multiply(x=w160, y=1000.0) -> (x*y=w169:dbl)
        n85 = Subtract(x=w169, y=w170) -> (x-y=w163:dbl)
        n86 = Less Or Equal To 0?(x=w163) -> (x <= 0?=w165:bool)
        n87 = Max & Min(x=w163, y=50.0) -> (min(x,y)=w161:dbl)  [unwired: 1 out]
      }
      frame "Reserve" {
        w171 = 0.0  # Don't move motors while reserved
        w173 = -1.0  # Infinite
        # "If loop needs to poll sensors or other\nvalues, use a timeout value. -1 waits for\nnext command to be sent."
      }
      frame "Read Current" {
        (unwired) 0.0 ("output")
      }
      frame "Drive for Distance" {
        n88 = Unbundle(w194) -> ("Iterations"=w193:i32)  [unwired: 1 out]
        n89 = Equal?(x=w193, y=0) -> (x = y?=w178:bool)
        n90 = local read "Gains"() -> (w180:T1)
        n91 = global read "Constants.vi" "Track Width"() -> (w179:dbl)
        n92 = Unbundle(w181) -> ("dx/dt"=w187:dbl, "dx/dt"=w186:dbl, "Yaw"=w185:dbl, w184:cluster{dbl, dbl})
        n93 = Bundle(cluster=T33 {"LeftDistance"=0.0, "RightDistance"=0.0, "LeftVelocity"=0.0, "RightVelocity"=0.0, "Angle"=0.0, "Location"={0.0, 0.0}} ("SensorData"), "LeftVelocity"=w187, "RightVelocity"=w186, "Angle"=w185, "Location"=w184) -> (w182:T33)  [unwired: 2 in]
        n94 = call "DriveForDistanceController.vi"("Distance"=w177, "MaxVel"="MaxVelDistance", "MaxAccel"="MaxAccelDistance", "Angle"=w176, "SensorData"=w182, "Gains"=w180, "Trackwidth"=w179, "Reset"=w178) -> ("Left Speed"=w191:dbl, "Right Speed"=w190:dbl, "Done"=w189:bool, "Time Left"=w188:dbl)  [unwired: 3 in, 1 out]
      }
      frame "Drive To Cube" {
        n95 = disable-structure shown="Enabled" {
          disable-tunnel: [w252 w297] -> w207
          disable-tunnel: [20.0 ("Infinite") 20.0 ("Infinite")] -> w206
          disable-tunnel: w205 -> [w250 _]
          disable-tunnel: w204 -> [w247 _]
          disable-tunnel: w203 -> [w243 _]
          disable-tunnel: w202 -> [w236 _]
          disable-tunnel: w201 -> [w235 _]
          disable-tunnel: w200 -> [w234 _]
          disable-tunnel: w199 -> [w233 _]
          disable-tunnel: [w232 w311] -> w198
          disable-tunnel: [w231 w312] -> w197
          disable-tunnel: w196 -> [w227 _]
          disable-tunnel: w195 -> [w222 _]
          frame Enabled {
            n96 = call <vilib>:"WPI_EncoderGet.vi"("EncoderDevRef"=w250) -> ("Distance"=w240:dbl)  [unwired: 5 in, 5 out]
            n97 = call <vilib>:"WPI_EncoderGet.vi"("EncoderDevRef"=w236) -> ("Distance"=w213:dbl)  [unwired: 5 in, 5 out]
            n98 = Unbundle(w243) -> ("Iterations"=w242:i32)  [unwired: 1 out]
            n99 = Greater Than 0?(x=w235) -> (x > 0?=w246:bool)
            n100 = Add(x=w234, y=w235) -> (x+y=w212:dbl)
            n101 = Equal?(x=w242, y=0) -> (x = y?=w225:bool)
            n102 = global read "Drive Published Globals.vi" "Data"() -> (w230:T28)
            n103 = Add(x=w247, y=w235) -> (x+y=w239:dbl)
            n104 = Unbundle By Name(w230) -> ("Timestamp"=w218:u32, "X"=w229:i32)
            n105 = Tick Count (ms)() -> (millisecond timer value=w217:u32)
            n106 = Subtract(x=w217, y=w218) -> (x-y=w216:u32)
            n107 = Less Or Equal?(x=w216, y=u32 300) -> (x <= y?=w214:bool)
            n108 = feedback #2(w227) -> (w223:dbl)
            n109 = case shown="True" w225 {
              tunnel: [w264 w265] -> w224
              tunnel: w223 -> [w264 _]
              tunnel: w222 -> [_ w265]
              frame False {
              }
              frame True {
              }
            }
            n110 = call <vilib>:"Get_YPRHfH.vi"("Device Number"=FRIC_navX_DeviceNumbersTypeDef."Dev0") -> ("YRPHfH"=w228:T30)  [unwired: 10 in]
            n111 = case shown="False" w246 {
              tunnel: w240 -> [w282 w290]
              tunnel: w239 -> [w283 w289]
              tunnel: [w280 w284] -> w252
              tunnel: w212 -> [w278 w288]
              tunnel: w213 -> [w279 w287]
              frame False {
                n112 = Less?(x=w279, y=w278) -> (x < y?=w277:bool)
                n113 = Less?(x=w282, y=w283) -> (x < y?=w281:bool)
                n114 = Or(x=w281, y=w277) -> (x .or. y?=w280:bool)
              }
              frame True {
                n115 = Greater?(x=w290, y=w289) -> (0:w286:bool)
                n116 = Greater?(x=w287, y=w288) -> (0:w285:bool)
                n117 = Or(x=w286, y=w285) -> (x .or. y?=w284:bool)
              }
            }
            n118 = Unbundle By Name(w228) -> ("Yaw"=w255:dbl)
            n119 = Subtract(x=w240, y=w239) -> (x-y=w238:dbl)
            n120 = Subtract(x=w213, y=w212) -> (x-y=w211:dbl)
            n121 = Absolute Value(x=w238) -> (abs(x)=w210:dbl)
            n122 = Absolute Value(x=w211) -> (abs(x)=w209:dbl)
            n123 = Max & Min(x=w210, y=w209) -> (min(x,y)=w208:dbl)  [unwired: 1 out]
            n124 = case shown="True" w214 {
              tunnel: w229 -> [_ w272]
              tunnel: w224 -> [w266 _]
              tunnel: w228 -> [_ w274]
              tunnel: [w266 w273] -> w226
              tunnel: w208 -> [_ w267]
              frame False {
              }
              frame True {
                n125 = To Double Precision Float(number=w272) -> (double precision float=w271:dbl)
                n126 = Unbundle By Name(w274) -> ("Yaw"=w275:dbl)
                n127 = call "LinearInterpolate.vi"("Points"="PixyCenteringValues", "Value"=w267) -> ("Output"=w270:dbl)  [unwired: 9 in]
                n128 = Subtract(x=w271, y=w270) -> (x-y=w269:dbl)
                n129 = expression code="x/320*50.0"(w269) -> (w276:dbl)
                n130 = Add(x=w276, y=w275) -> (x+y=w273:dbl)
              }
            }
            n131 = feedback-in #2(w226) -> ()
            n132 = Subtract(x=w226, y=w255) -> (x-y=w254:dbl)
            n133 = Add(x=w254, y=180.0) -> (x+y=w259:dbl)
            n134 = Quotient & Remainder(x=w259, y=360.0) -> (x-y*floor(x/y)=w257:dbl)  [unwired: 1 out]
            n135 = Less?(x=w210, y=60.0) -> ()  [unwired: 1 out]
            n136 = Subtract(x=w257, y=180.0) -> (x-y=w253:dbl)
            n137 = Equal?(x=0.0, y=w253) -> (x = y?=w262:bool)
            n138 = call "LinearInterpolate.vi"("Points"=cluster{"X":dbl, "Y":dbl}[] [{"X"=0.0, "Y"=0.0}, {"X"=0.02, "Y"=0.0}, {"X"=0.021, "Y"=0.19}, {"X"=1.0, "Y"=1.0}], "Value"=w233) -> ("Output"=w245:dbl)  [unwired: 9 in]
            n139 = case shown="False" w262 {
              tunnel: [w291 0.0] -> w220
              tunnel: w253 -> [w292 _]
              frame False {
                n140 = call-poly <vilib>:"PID.vi"("output range"=cluster{"output high":dbl, "output low":dbl} {"output high"=0.6, "output low"=-0.6}, "PID gains"=T35 {"proportional gain (Kc)"=0.1, "integral time (Ti, min)"=0.0, "derivative time (Td, min)"=0.0}, "process variable"=w292, "setpoint"=0.0) -> ("output"=w291:dbl)  [unwired: 6 in, 1 out]
              }
              frame True {
              }
            }
            n141 = call "LinearInterpolate.vi"("Points"=cluster{"X":dbl, "Y":dbl}[] [{"X"=0.0, "Y"=0.0}, {"X"=0.01, "Y"=0.0}, {"X"=0.011, "Y"=0.1}, {"X"=1.0, "Y"=1.0}], "Value"=w220) -> ("Output"=w219:dbl)  [unwired: 9 in]
            n142 = call <vilib>:"WPI_JoystickArcadeMapping.vi"("Max Output"=1.0, "Square Inputs"=FALSE, "Y axis value"=w245, "X axis value"=w219) -> ("Right Motor Value"=w231:dbl, "Left Motor Value"=w232:dbl)  [unwired: 6 in]
          }
          frame Disabled {
            w315 = 0.1 ("lower limit")
            # "Speed"
            n143 = global read "Drive Published Globals.vi" "Data"() -> (w310:T28)
            n144 = Unbundle By Name(w310) -> ("X"=w309:i32, "Y"=w301:i32, "Width"=w306:i32, "Height"=w305:i32)
            n145 = Multiply(x=w306, y=w305) -> (x*y=w300:i32)
            n146 = Subtract(x=w309, y="CenterSetpoint") -> (x-y=w308:i32)
            n147 = call "derivative.vi"("Starting value"=w308, "x"=w308) -> ("dx/dt"=w307:dbl)  [unwired: 9 in]
            n148 = Subtract(x="AreaSetpoint", y=w300) -> (x-y=w322:i32)
            n149 = Multiply(x=w308, y="KpX") -> (x*y=w319:dbl)
            n150 = Multiply(x=w307, y="KdX") -> (x*y=w318:dbl)
            n151 = Less Or Equal?(x=w301, y="MaxY") -> (x <= y?=w298:bool)
            n152 = Multiply(x=w322, y="KpY") -> (x*y=w323:dbl)
            n153 = Add(x=w319, y=w318) -> (x+y=w320:dbl)
            n154 = Subtract(x=w319, y=w318) -> (x-y=w317:dbl)
            n155 = Add(x=w323, y=w320) -> (x+y=w325:dbl)
            n156 = Subtract(x=w323, y=w317) -> (x-y=w324:dbl)
            n157 = Greater Or Equal?(x=w300, y="EndCondArea") -> (x >= y?=w299:bool)
            n158 = In Range and Coerce(upper limit="MaxSpeed", x=w325, lower limit=w315) -> (coerced(x)=w311:dbl)  [unwired: 1 out]
            n159 = In Range and Coerce(upper limit="MaxSpeed", x=w324, lower limit=w315) -> (coerced(x)=w312:dbl)  [unwired: 1 out]
            n160 = And(x=w298, y=w299) -> (x .and. y?=w297:bool)
          }
        }
      }
      frame "Turn to Angle" {
        n161 = Unbundle(w340) -> ("Iterations"=w339:i32)  [unwired: 1 out]
        n162 = Equal To 0?(x=w339) -> (x = 0?=w337:bool)
        n163 = call <vilib>:"Get_YPRHfH.vi"("Device Number"=FRIC_navX_DeviceNumbersTypeDef."Dev0") -> ("YRPHfH"=w336:T30)  [unwired: 10 in]
        n164 = Unbundle By Name(w336) -> ("Yaw"=w335:dbl)
        n165 = call "TurnToAngleController.vi"("MaxAccel"="MaxAccelAngle", "MaxVel"="MaxVelAngle", "Reset"=w337, "Gains"="TurnToAngleGains", "CurrentAngle"=w335, "TargetAngle"=w338) -> ("Done"=w328:bool, "Time Left"=w329:u32, "RightPower"=w330:dbl, "LeftPower"=w331:dbl)  [unwired: 2 out]
      }
      frame "Arc Turn" {
        n166 = Add(x=w346, y=w345) -> (x+y=w353:dbl)
        n167 = call <vilib>:"Get_YPRHfH.vi"("Device Number"=FRIC_navX_DeviceNumbersTypeDef."Dev0") -> ("YRPHfH"=w349:T30)  [unwired: 10 in]
        n168 = Unbundle By Name(w349) -> ("Yaw"=w347:dbl)
        n169 = Subtract(x=w347, y=w353) -> (x-y=w355:dbl)
        n170 = Add(x=w355, y=180.0) -> (x+y=w358:dbl)
        n171 = Quotient & Remainder(x=w358, y=360.0) -> (x-y*floor(x/y)=w356:dbl)  [unwired: 1 out]
        n172 = Subtract(x=w356, y=180.0) -> (x-y=w352:dbl)
        n173 = In Range and Coerce(upper limit=1.0, x=w352, lower limit=-1.0) -> ()  [unwired: 2 out]
        n174 = call-poly <vilib>:"PID.vi"("output range"=cluster{"output high":dbl, "output low":dbl} {"output high"=0.5, "output low"=-0.5}, "PID gains"=T35 {"proportional gain (Kc)"=0.02, "integral time (Ti, min)"=0.0, "derivative time (Td, min)"=0.0}, "process variable"=w352, "setpoint"=0.0) -> ("output"=w343:dbl)  [unwired: 6 in, 1 out]
      }
      frame "Drive Path" {
        n175 = global read "Constants.vi" "Track Width"() -> (w365:dbl)
        n176 = Unbundle(w370) -> ("dx/dt"=w374:dbl, "dx/dt"=w373:dbl, "Yaw"=w372:dbl, w371:cluster{dbl, dbl})
        n177 = Unbundle(w366) -> ("Iterations"=w367:i32)  [unwired: 1 out]
        n178 = Equal To 0?(x=w367) -> (x = 0?=w368:bool)
        n179 = Bundle(cluster=T33 {"LeftDistance"=0.0, "RightDistance"=0.0, "LeftVelocity"=0.0, "RightVelocity"=0.0, "Angle"=0.0, "Location"={0.0, 0.0}} ("SensorData"), "LeftVelocity"=w374, "RightVelocity"=w373, "Angle"=w372, "Location"=w371) -> (w375:T33)  [unwired: 2 in]
        n180 = call "PurePursuit.vi"("RobotNeededPathData"=w379, "SensorData"=w375, "Trackwidth"=w365, "Reset"=w368, "Gains"="Gains") -> ("LeftValue"=w378:dbl, "RightValue"=w377:dbl, "Done"=w376:bool)  [unwired: 6 in, 2 out]
      }
    }
    n181 = call "Drive Check for New Command.vi"("input cluster"=w137, "Wait time (ms)"=w143, "Finished?"=w142) -> ("Completion"=w145:T5, "Subsystem Name"=w139:string, "Current Command"=w140:T2, "Initial Trace String"=w141:string, "Next Command"=w144:T37)  [unwired: 4 in]
    n182 = Bundle("LeftValue"=w118, "RightValue"=w117) -> (→"Setpoints":cluster{"LeftValue":dbl, "RightValue":dbl})  [unwired: 1 in]
    n183 = global write "Drive Published Globals.vi" "MotorRight"(w117) -> ()
    n184 = global write "Drive Published Globals.vi" "MotorLeft"(w118) -> ()
    n185 = case shown="\"Successful\", \"Aborted\"" w145 {
      selector: w145 -> [_ w388]
      tunnel: w141 -> [_ w383]
      tunnel: w140 -> [_ w384]
      tunnel: w139 -> [_ w380]
      frame "Incomplete", Default {
        # "Continuing current command"
      }
      frame "Successful", "Aborted" {
        # "Report and setup for next command"
        n186 = Unbundle By Name(w384) -> ("Left Speed"=w386:dbl, "Right Speed"=w387:dbl, "Duration"=w381:dbl)
        n187 = Format Into String(format string="L %.1f, R %.1f, D %f", initial string=w383, w386, w387, w381) -> (resulting string=w382:string)  [unwired: 1 in, 1 out]
        "Current\nCmd" <- w382
        n188 = call <vilib>:"Trace Results.vi"("Status of previous command"=w388, "Description"=w382, "Subsystem"=w380) -> ()  [unwired: 9 in]
      }
    }
    n189 = call <vilib>:"WPI_RobotDriveMotors.vi"("RightSpeed"=w117, "LeftSpeed"=w118, "RobotDriveDevRef"=w123) -> ()  [unwired: 1 in, 8 out]
    n190 = call <vilib>:"WPI_RobotDriveMotors.vi"("RightSpeed"=w117, "LeftSpeed"=w118, "RobotDriveDevRef"=w122) -> ()  [unwired: 1 in, 8 out]
  }
  n191 = while {
    tunnel: w20 -> [w390]
    stop <- FALSE stop-if-true
    n192 = call "Drive Controller Interactive Check.vi"("Interactive Command In"="Interactive Values", "Default Command"=w390, "Buttons"="Buttons") -> ("Interactive Command Out"=w392:T2, "Trace String"=w393:string, "Schedule"=w394:bool)  [unwired: 6 in]
    n193 = case shown="False" w394 {
      tunnel: [w403 w411] -> w395
      tunnel: [w402 w407] -> w396
      tunnel: w393 -> [_ w409]
      tunnel: w392 -> [_ w408]
      frame False {
        n194 = Tick Count (ms)() -> (millisecond timer value=w406:u32)
        n195 = call "Read Drive Operation.vi"() -> ("Command Info"=w400:T25, "SubSystem Data"=w399:T2)  [unwired: 9 in, 1 out]
        n196 = Unbundle(w399) -> ("Operation"=w404:T3, "Left Speed"=w401:dbl)  [unwired: 9 out]
        n197 = Unbundle(w400) -> ("Status"=w403:T5)  [unwired: 2 out]
        n198 = Subtract(x=w406, y=w404) -> (x-y=w405:u32)
        n199 = Bundle(w405, "Left Speed"=w401) -> (w402:cluster{u32, "Left Speed":dbl})  [unwired: 1 in]
      }
      frame True {
        n200 = call "Drive Command Helper.vi"("Description"=w409, "SubSystem Data"=w408) -> ("Command Info Out"=w410:T25, "Command Timing"=w407:cluster{"Start Time (ms)":u32, "Iterations":i32})  [unwired: 7 in, 1 out]
        n201 = Unbundle(w410) -> ("Status"=w411:T5)  [unwired: 2 out]
      }
    }
    "Status" <- w395
    "Command Timing" <- w396
    n202 = Wait (ms)(milliseconds to wait=u32 20) -> ()  [unwired: 1 out]
  }
